vi "disconnect.vi"(8 "error in (no error)":errorcluster, 11 "MyComics.org_class in":refnum<class "MyComics.org_class.lvclass">) -> (0 "error out":errorcluster, 3 "MyComics.org_class out":refnum<class "MyComics.org_class.lvclass">)   [LabVIEW 2024, in "MyComics.org_class.lvclass"]
uses:
  MyComics.org_class.lvclass
  MyComics.org_class.lvclass/MyComics.org_class.ctl
  <vilib>/httpClient/LabVIEWHTTPClient.lvlib
  <vilib>/httpClient/ClientHandle.ctl
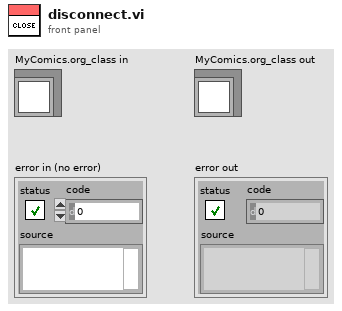
[diagram p1: front panel]
types:
  T1 = typedef "LabVIEWHTTPClient.lvlib/ClientHandle.ctl" = refnum<k1>
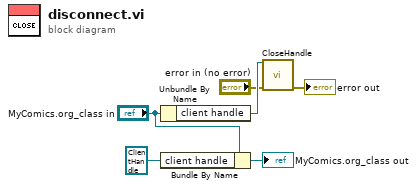
[diagram p0: block diagram]
diagram:
  n1 = Unbundle By Name("MyComics.org_class in") -> ("client handle"=w6:T1)
  n2 = Bundle By Name(cluster="MyComics.org_class in", "client handle"=T1 refnum) -> (→"MyComics.org_class out":refnum<class "MyComics.org_class.lvclass">)
  n3 = call <vilib>:"CloseHandle.vi"("client handle"=w6, "error in (no error)"="error in (no error)") -> ("error out"=→"error out":errorcluster)  [unwired: 13 in]
